vi "AplicaPond_C_RefAcusticaCAM.vi"(1 "result":string[][](array[string])) -> (0 "output array":string[][](array[string]))   [LabVIEW 2019, in "Prueba031.lvclass"]
doc: "Este SubVI lee la curva de referencia en dB desde el certificado de calibracion del CAM\npara los ensayos que usan generador interno."
uses:
  Prueba031.lvclass
panel:
  out "114db(C)":string[](array[string])
  out "94db(C)":string[](array[string])
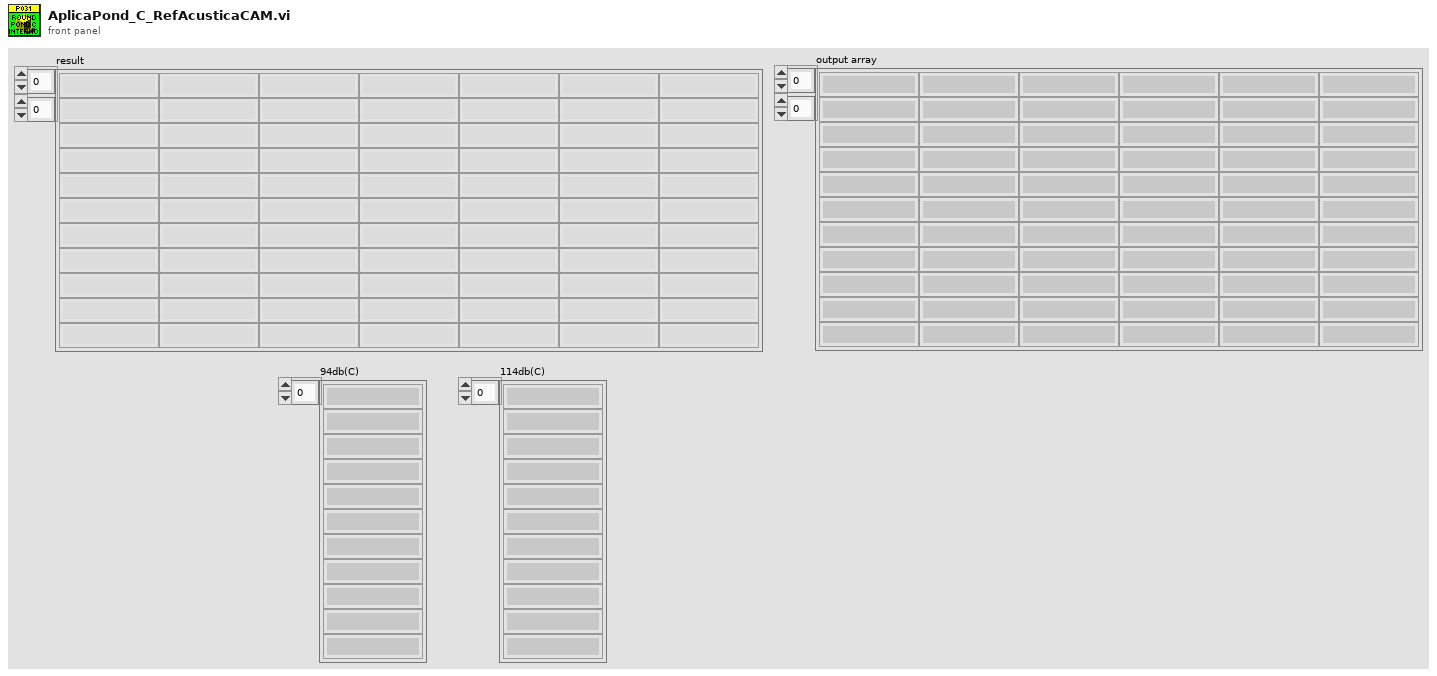
[diagram p1: front panel]
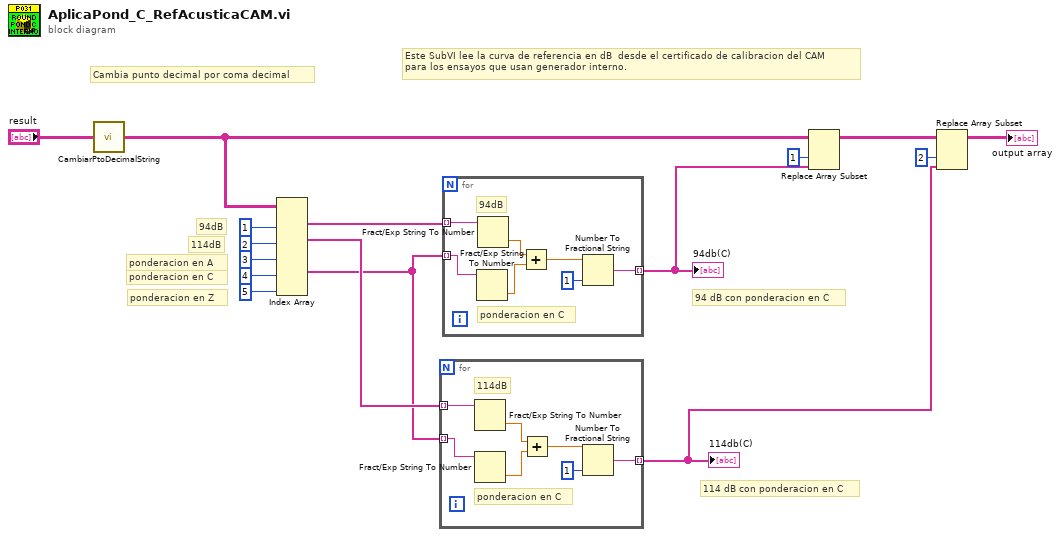
[diagram p0: block diagram]
diagram:
  # "114 dB con ponderacion en C"
  # "94 dB con ponderacion en C"
  # "ponderacion en Z"
  # "ponderacion en C"
  # "ponderacion en A"
  # "114dB"
  # "94dB"
  # "Este SubVI lee la curva de referencia en dB  desde el certificado de calibracion del CAM\npara los ensayos que usan generador interno."
  # "Cambia punto decimal por coma decimal"
  n1 = call "CambiarPtoDecimalString.vi"("result"="result") -> ("result out"=w1:string[][])
  n2 = Index Array(array=w1, index (col) #1=1 ("disabled index (col)"), index (col) #2=2 ("disabled index (row)"), index (col) #3=3 ("index (col)"), index (col) #4=4 ("index (col)"), index (col) #5=5 ("index (col)")) -> (element #1=w7:string[], element #2=w6:string[], element #4=w5:string[])  [unwired: 5 in, 2 out]
  n3 = for {
    tunnel: w6 -> [w23] mode=indexing
    tunnel: [w21] -> w10 mode=indexing
    tunnel: w5 -> [w20] mode=indexing
    # "ponderacion en C"
    # "114dB"
    n4 = Fract/Exp String To Number(string=w23) -> (number=w18:dbl)  [unwired: 3 in, 1 out]
    n5 = Fract/Exp String To Number(string=w20) -> (number=w19:dbl)  [unwired: 3 in, 1 out]
    n6 = Add(x=w18, y=w19) -> (x+y=w17:dbl)
    n7 = Number To Fractional String(number=w17, precision (6)=i16 1) -> (F-format string=w21:string)  [unwired: 2 in]
  }
  "114db(C)" <- w10
  n8 = for {
    tunnel: w7 -> [w30] mode=indexing
    tunnel: [w28] -> w11 mode=indexing
    tunnel: w5 -> [w27] mode=indexing
    # "ponderacion en C"
    # "94dB"
    n9 = Fract/Exp String To Number(string=w27) -> (number=w25:dbl)  [unwired: 3 in, 1 out]
    n10 = Fract/Exp String To Number(string=w30) -> (number=w26:dbl)  [unwired: 3 in, 1 out]
    n11 = Add(x=w26, y=w25) -> (x+y=w24:dbl)
    n12 = Number To Fractional String(number=w24, precision (6)=i16 1) -> (F-format string=w28:string)  [unwired: 2 in]
  }
  "94db(C)" <- w11
  n13 = Replace Array Subset(array=w1, new element=w11, index (col)=1 ("disabled index (col)")) -> (w12:string[][])  [unwired: 1 in]
  n14 = Replace Array Subset(array=w12, new element=w10, index (col)=2 ("disabled index (col)")) -> (→"output array":string[][])  [unwired: 1 in]
